vi "New Client.vi"(5 "Realm":string, 7 "Address":string, 11 "error in (no error)":errorcluster) -> (4 "reference out":refnum<class "WAMP Client.lvclass">, 15 "error out":errorcluster)   [LabVIEW 2020, in "wamplv.lvlib" / "WAMP Client.lvclass"]
uses:
  WAMP Client.lvclass
  WAMP Client.lvclass/WAMP Client.ctl
  Comm Handlers/Websocket Handler/Websocket Handler.lvclass
  <vilib>/LabVIEW Open Source Project/OpenURI/uri/URI.lvclass
  Comm Handlers/RawSocket Handler/RawSocket Handler.lvclass
  <vilib>/ErrorRing/Error Ring.xnode
  <vilib>/Utility/error.llb/Error Cluster From Error Code.vi
  C:/local/wamplv/Comm Handlers/CommHandlerBase/CommHandlerBase.lvclass
  C:/local/wamplv/Comm Handlers/ICommHandler/ICommHandler.lvclass
  C:/local/wamplv/Comm Handlers/RawSocket Handler/RawSocket Handler.lvclass
  C:/local/wamplv/Comm Handlers/Websocket Handler/Websocket Handler.lvclass
  Comm Handlers/CommHandlerBase/CommHandlerBase.lvclass
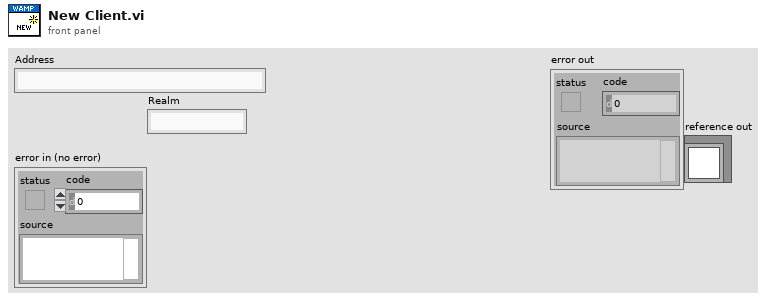
[diagram p1: front panel]
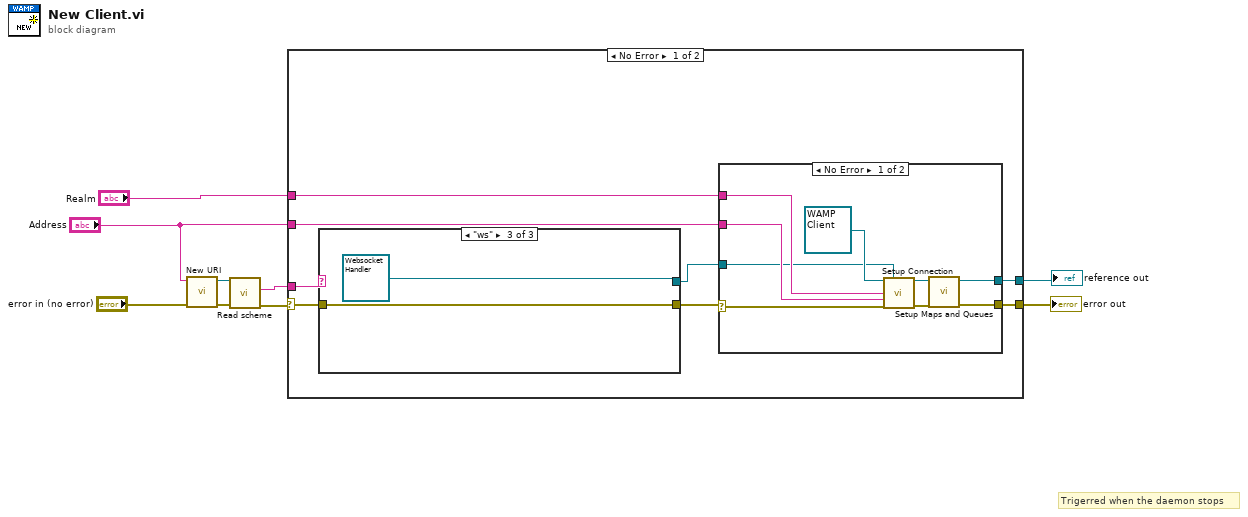
[diagram p0: block diagram]
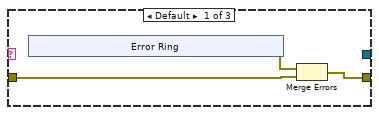
[diagram p3: hidden frame]
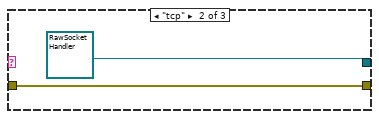
[diagram p4: hidden frame]
diagram:
  # "Trigerred when the daemon stops"
  n1 = call <vilib>:"New URI.vi"("error in (no error)"="error in (no error)", "URI"="Address") -> ("error out"=w4:errorcluster, "URI"=w5:refnum<class "URI.lvclass">)  [unwired: 8 in]
  n2 = call <vilib>:"Read scheme.vi"("error in (no error)"=w4, "URI in"=w5) -> ("error out"=w3:errorcluster, "scheme"=w2:string)  [unwired: 7 in, 1 out]
  n3 = case shown="No Error" w3 {
    selector: w3 -> [w12 w39]
    tunnel: "Realm" -> [w17 _]
    tunnel: [w16 _] -> w1
    tunnel: [w15 w39] -> w7
    tunnel: "Address" -> [w14 _]
    tunnel: w2 -> [w13 _]
    frame No Error {
      n4 = case shown="\"ws\"" w13 {
        tunnel: [_ refnum<class "RawSocket Handler.lvclass"> refnum ("wamplv.lvlib:RawSocket Handler.lvclass") refnum<class "Websocket Handler.lvclass"> refnum ("Websocket Handler.lvclass")] -> w11
        tunnel: w12 -> [w29 w35 w37]
        tunnel: [w30 w35 w37] -> w10
        frame Default {
          n5 = xnode "Error Ring"() -> ("error out"=w28:errorcluster)
          n6 = Merge Errors(w28, w29) -> (w30:errorcluster)
        }
        frame "tcp" {
        }
        frame "ws" {
        }
      }
      n7 = case shown="No Error" w10 {
        selector: w10 -> [w18 w27]
        tunnel: w17 -> [w26 _]
        tunnel: [w23 _] -> w16
        tunnel: [w22 w27] -> w15
        tunnel: w14 -> [w20 _]
        tunnel: w11 -> [w19 _]
        frame No Error {
          n8 = call-dynamic "Setup Connection.vi"("WAMP Client in"=refnum<class "WAMP Client.lvclass"> refnum ("WAMP Client.lvclass"), "ICommHandler.lvclass"=w19, "Realm"=w26, "Address"=w20, "error in (no error)"=w18) -> ("WAMP Client out"=w24:refnum<class "WAMP Client.lvclass">, "error out"=w21:errorcluster)  [unwired: 9 in]
          n9 = call-dynamic "Setup Maps and Queues.vi"("error in (no error)"=w21, "WAMP Client in"=w24) -> ("error out"=w22:errorcluster, "WAMP Client out"=w23:refnum<class "WAMP Client.lvclass">)  [unwired: 8 in]
        }
        frame Error {
        }
      }
    }
    frame Error {
    }
  }
  "error out" <- w7
  "reference out" <- w1
